vi "n分频.vi"(8 "error in":errorcluster, 10 "preset value":u32=10, 11 "count down":bool) -> (0 "error out":errorcluster, 2 "counter value":u32, 3 "Q":bool)   [LabVIEW 2012]
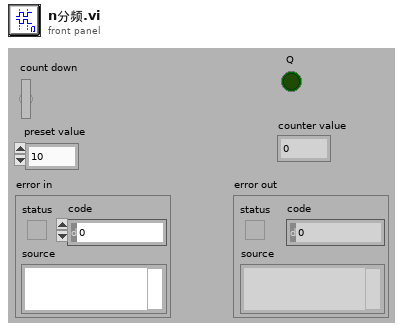
[diagram p1: front panel]
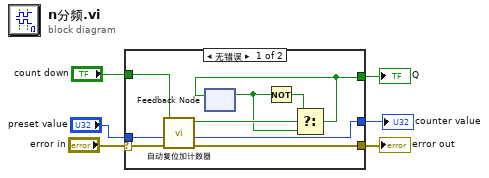
[diagram p0: block diagram]
diagram:
  n1 = case shown="无错误" "error in" {
    selector: "error in" -> [w9 w16]
    tunnel: [w8 w16] -> w5
    tunnel: "count down" -> [w15 _]
    tunnel: "preset value" -> [w14 _]
    tunnel: [w12 _] -> w2
    tunnel: [w7 _] -> w1
    frame No Error {
      n2 = call "自动复位加计数器.vi"("error in"=w9, "preset value"=w14, "count up"=w15) -> ("error out"=w8:errorcluster, "counter value"=w7:u32, "done"=w13:bool)  [unwired: 6 in]
      n3 = feedback #1() -> (w11:bool)  [unwired: 1 in]
      n4 = Not(x=w11) -> (.not. x?=w10:bool)
      n5 = Select(t=w10, s=w13, f=w11) -> (s? t:f=w12:bool)
      n6 = feedback-in #1(w12) -> ()
    }
    frame Error {
    }
  }
  "error out" <- w5
  "Q" <- w2
  "counter value" <- w1
